vi "test_libssh2_sftp_fstatvfs.vi"() -> ()   [LabVIEW 2013, in "libssh2_integration_tests.lvlib"]
uses:
  libssh2_integration_tests.lvlib
  <vilib>/addons/_JKI Toolkits/Caraya/classes/Test/Test.lvclass
  libssh2/libssh2.lvlib
  <vilib>/addons/_JKI Toolkits/Caraya/classes/Assert/Assert.lvclass
panel:
  out "error out":errorcluster
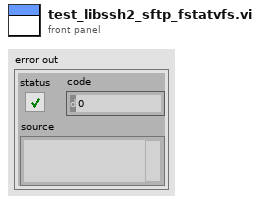
[diagram p1: front panel]
types:
  T1 = typedef "libssh2.lvlib/Session Refnum.ctl" = refnum<k1>
  T2 = typedef "libssh2.lvlib/SFTP Refnum.ctl" = refnum<k1>
  T3 = typedef "libssh2.lvlib/SFTP Handle Refnum.ctl" = refnum<k1>
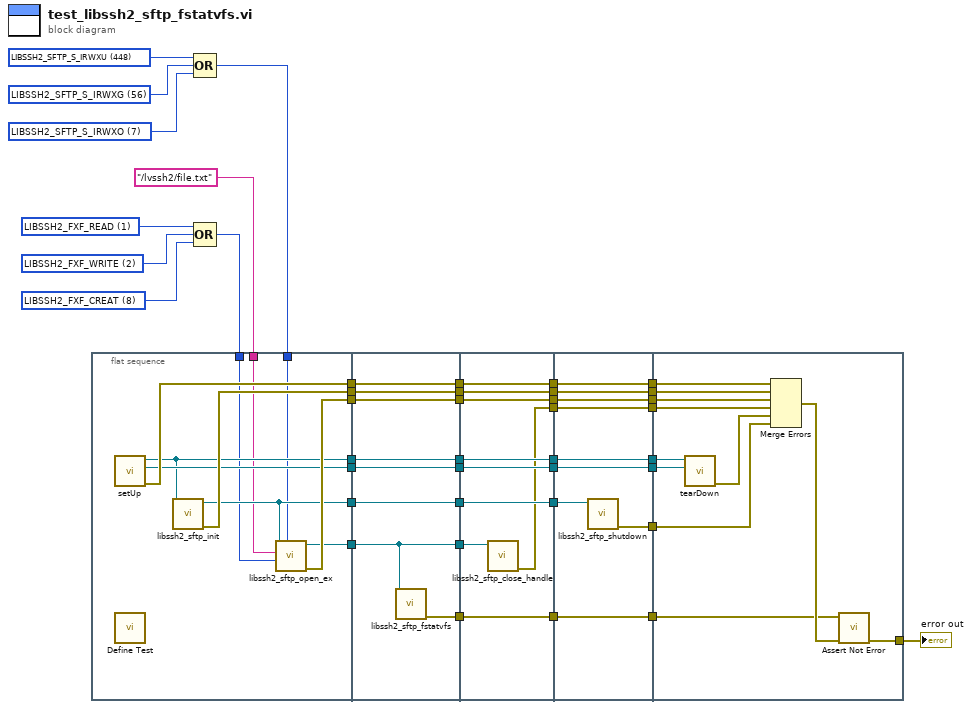
[diagram p0: block diagram]
diagram:
  w37 = u32 2 items=["LIBSSH2_FXF_READ"=1, "LIBSSH2_FXF_WRITE"=2, "LIBSSH2_FXF_APPEND"=4, "LIBSSH2_FXF_CREAT"=8, "LIBSSH2_FXF_TRUNC"=16, "LIBSSH2_FXF_EXCL"=32] ("flags")
  w38 = u32 1 items=["LIBSSH2_FXF_READ"=1, "LIBSSH2_FXF_WRITE"=2, "LIBSSH2_FXF_APPEND"=4, "LIBSSH2_FXF_CREAT"=8, "LIBSSH2_FXF_TRUNC"=16, "LIBSSH2_FXF_EXCL"=32] ("flags")
  w36 = u32 8 items=["LIBSSH2_FXF_READ"=1, "LIBSSH2_FXF_WRITE"=2, "LIBSSH2_FXF_APPEND"=4, "LIBSSH2_FXF_CREAT"=8, "LIBSSH2_FXF_TRUNC"=16, "LIBSSH2_FXF_EXCL"=32] ("flags")
  w39 = 7 items=["LIBSSH2_SFTP_S_IRWXU"=448, "LIBSSH2_SFTP_S_IRUSR"=256, "LIBSSH2_SFTP_S_IWUSR"=128, "LIBSSH2_SFTP_S_IXUSR"=64, "LIBSSH2_SFTP_S_IRWXG"=56, "LIBSSH2_SFTP_S_IRGRP"=32, "LIBSSH2_SFTP_S_IWGRP"=16, "LIBSSH2_SFTP_S_IXGRP"=8, "LIBSSH2_SFTP_S_IRWXO"=7, "LIBSSH2_SFTP_S_IROTH"=4, "LIBSSH2_SFTP_S_IWOTH"=2, "LIBSSH2_SFTP_S_IXOTH"=1] ("mode")
  w40 = 56 items=["LIBSSH2_SFTP_S_IRWXU"=448, "LIBSSH2_SFTP_S_IRUSR"=256, "LIBSSH2_SFTP_S_IWUSR"=128, "LIBSSH2_SFTP_S_IXUSR"=64, "LIBSSH2_SFTP_S_IRWXG"=56, "LIBSSH2_SFTP_S_IRGRP"=32, "LIBSSH2_SFTP_S_IWGRP"=16, "LIBSSH2_SFTP_S_IXGRP"=8, "LIBSSH2_SFTP_S_IRWXO"=7, "LIBSSH2_SFTP_S_IROTH"=4, "LIBSSH2_SFTP_S_IWOTH"=2, "LIBSSH2_SFTP_S_IXOTH"=1] ("mode")
  w41 = 448 items=["LIBSSH2_SFTP_S_IRWXU"=448, "LIBSSH2_SFTP_S_IRUSR"=256, "LIBSSH2_SFTP_S_IWUSR"=128, "LIBSSH2_SFTP_S_IXUSR"=64, "LIBSSH2_SFTP_S_IRWXG"=56, "LIBSSH2_SFTP_S_IRGRP"=32, "LIBSSH2_SFTP_S_IWGRP"=16, "LIBSSH2_SFTP_S_IXGRP"=8, "LIBSSH2_SFTP_S_IRWXO"=7, "LIBSSH2_SFTP_S_IROTH"=4, "LIBSSH2_SFTP_S_IWOTH"=2, "LIBSSH2_SFTP_S_IXOTH"=1] ("mode")
  n1 = flat-sequence {
    tunnel: [w51] -> w27
    tunnel: [w50] -> w26
    tunnel: [w49] -> w25
    tunnel: [w48] -> w24
    tunnel: [w47] -> w23
    tunnel: [w46] -> w22
    tunnel: [w42] -> w21
    tunnel: w6 -> [w43]
    tunnel: "/lvssh2/file.txt" ("filename") -> [w44]
    tunnel: w5 -> [w45]
    tunnel: w27 -> [w59]
    tunnel: [w59] -> w20
    tunnel: w26 -> [w58]
    tunnel: [w58] -> w19
    tunnel: w25 -> [w57]
    tunnel: [w57] -> w18
    tunnel: w24 -> [w56]
    tunnel: [w56] -> w17
    tunnel: w23 -> [w55]
    tunnel: [w55] -> w16
    tunnel: w22 -> [w54]
    tunnel: [w54] -> w15
    tunnel: w21 -> [w53]
    tunnel: [w53] -> w14
    tunnel: [w52] -> w2
    tunnel: [w62] -> w7
    tunnel: w20 -> [w68]
    tunnel: [w68] -> w8
    tunnel: w19 -> [w67]
    tunnel: [w67] -> w9
    tunnel: w18 -> [w66]
    tunnel: [w66] -> w10
    tunnel: w17 -> [w65]
    tunnel: [w65] -> w11
    tunnel: w16 -> [w64]
    tunnel: [w64] -> w12
    tunnel: w15 -> [w63]
    tunnel: [w63] -> w13
    tunnel: w14 -> [w61]
    tunnel: [w60] -> w3
    tunnel: w2 -> [w60]
    tunnel: w13 -> [w77]
    tunnel: [w77] -> w35
    tunnel: w12 -> [w76]
    tunnel: [w76] -> w34
    tunnel: w11 -> [w73]
    tunnel: w10 -> [w75]
    tunnel: [w75] -> w33
    tunnel: w9 -> [w74]
    tunnel: [w74] -> w32
    tunnel: [w72] -> w31
    tunnel: w8 -> [w71]
    tunnel: [w71] -> w30
    tunnel: [w70] -> w29
    tunnel: w7 -> [w70]
    tunnel: [w69] -> w4
    tunnel: w3 -> [w69]
    tunnel: w35 -> [w88]
    tunnel: w34 -> [w87]
    tunnel: w33 -> [w86]
    tunnel: w32 -> [w83]
    tunnel: w31 -> [w82]
    tunnel: w30 -> [w81]
    tunnel: w29 -> [w80]
    tunnel: w4 -> [w79]
    tunnel: [w78] -> w1
    frame #0 {
      n2 = call "setUp.vi"() -> ("error out"=w49:errorcluster, "connection ID"=w47:refnum<k5>, "session"=w46:T1)  [unwired: 9 in]
      n3 = call <vilib>:"Define Test.vi"() -> ()  [unwired: 10 in, 2 out]
      n4 = call "libssh2_sftp_init.vi"("session"=w46) -> ("error out"=w50:errorcluster, "sftp"=w48:T2)  [unwired: 9 in]
      n5 = call "libssh2_sftp_open_ex.vi"("mode"=w45, "flags"=w43, "filename"=w44, "sftp"=w48) -> ("error out"=w51:errorcluster, "sftp handle"=w42:T3)  [unwired: 6 in]
    }
    frame #1 {
      n6 = call "libssh2_sftp_fstatvfs.vi"("sftp handle"=w53) -> ("error out"=w52:errorcluster)  [unwired: 9 in, 1 out]
    }
    frame #2 {
      n7 = call "libssh2_sftp_close_handle.vi"("sftp handle"=w61) -> ("error out"=w62:errorcluster)  [unwired: 10 in]
    }
    frame #3 {
      n8 = call "libssh2_sftp_shutdown.vi"("sftp"=w73) -> ("error out"=w72:errorcluster)  [unwired: 10 in]
    }
    frame #4 {
      n9 = call "tearDown.vi"("connection ID"=w87, "session"=w88) -> ("error out"=w85:errorcluster)  [unwired: 9 in]
      n10 = Merge Errors(w86, w83, w81, w80, w85, w82) -> (w84:errorcluster)
      n11 = call <vilib>:"Assert Not Error.vi"("error in (no error)"=w84, "Not Error?"=w79) -> ("error out"=w78:errorcluster)  [unwired: 8 in, 1 out]
    }
  }
  n12 = Compound Arithmetic op=OR(w41, w40, w39) -> (w5:i32)
  n13 = Compound Arithmetic op=OR(w38, w37, w36) -> (w6:u32)
  "error out" <- w1
